vi "acquistion Real and Imaginary spectrum.vi"(4 "slope":i32(ring)=10280 items=["Rising"=10280, "Falling"=10171], 5 "maximum value":dbl=5.0, 6 "Triggering level":dbl format="%0.2f", 7 "minimum value":dbl=-5.0, 8 "error in":errorcluster, 9 "Sampling Frecuency (Hz)":dbl, 10 "Number of Samples":i32=-1, 11 "Analog In Channels":T4) -> (0 "error out":errorcluster, 3 "Data Read":waveform(dbl)[](graph))   [LabVIEW 2017]
uses:
  <vilib>/Analysis/4window.llb/windowTd.ctl
  <vilib>/DAQmx/read.llb/DAQmx Read (Analog 1D Wfm NChan NSamp).vi
  <vilib>/DAQmx/create/channels.llb/DAQmx Create Channel (AI-Voltage-Basic).vi
  <vilib>/DAQmx/configure/timing.llb/DAQmx Timing (Use Waveform).vi
  <vilib>/DAQmx/configure/trigger.llb/DAQmx Start Trigger (Analog Edge).vi
  <vilib>/DAQmx/miscellaneous.llb/DAQmx Fill In Error Info.vi
  <vilib>/measure/maspectr.llb/FFT Spectrum (Real-Im) for N Chan.vi
  <instrlib>/NI USB-6356/NI USB-6356.lvlib
  <vilib>/Analysis/NI_AALPro.lvlib
  <vilib>/measure/NI_MAPro.lvlib
panel:
  in  "window parameter":dbl=nan
  out "Real Part 2":T1(graph)
  out "Imaginary Part":T2(graph)
  in  "gain":dbl=1.0 min=1.0
  in  "Use Trigger?":bool
  out "Real Part":cluster{"f0":dbl, "df":dbl, "magnitude":dbl[]}(graph)
  out "averages completed":dbl
  out "averaging done":bool
  in  "averaging parameters":T3={"averaging mode"=enum."Vector averaging", "weighting mode"=enum."Exponential", "number of averages"=10} {"number of averages" min=1}
  in  "restart averaging (F)":bool
  in  "Channel Trigger":u16(ring) items=["ai0", "ai1", "ai2", "ai3", "ai4", "ai5", "ai6", "ai7"]
  in  "Stop Process":bool
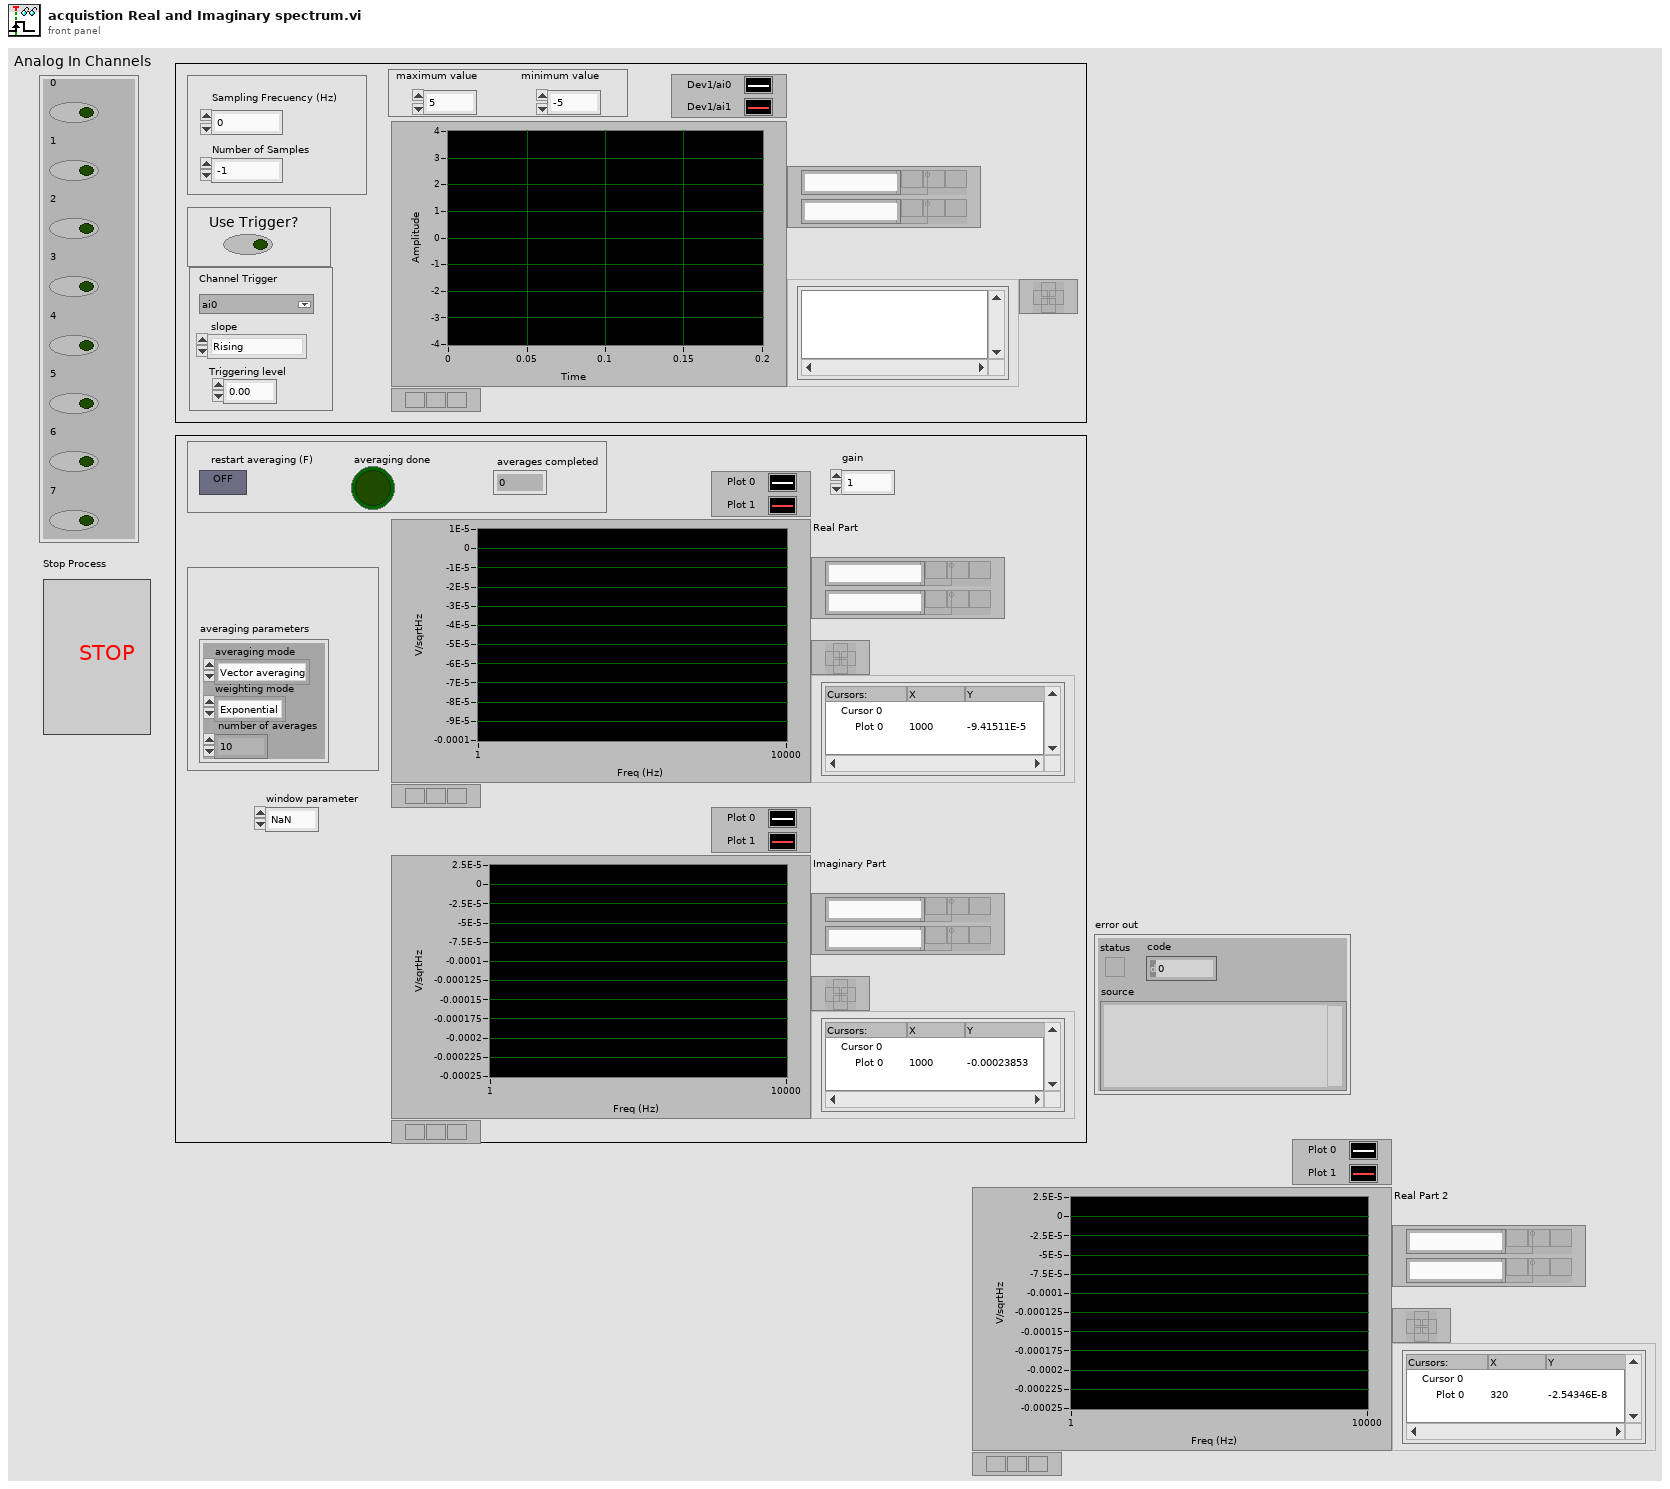
[diagram p1: front panel]
types:
  T1 = cluster{"f0":dbl, "df":dbl, "imaginary part":dbl[]}[]
  T2 = cluster{"f0":dbl, "df":dbl, "imaginary part":dbl[]}
  T3 = cluster{"averaging mode":enum16{"No averaging", "Vector averaging", "RMS averaging", "Peak hold"}, "weighting mode":enum16{"Linear", "Exponential"}, "number of averages":u32}
  T4 = cluster{"0":bool, "1":bool, "2":bool, "3":bool, "4":bool, "5":bool, "6":bool, "7":bool}
  T5 = typedef "NI_AALPro.lvlib/windowTd.ctl" = u32
  T6 = enum8{"Enabled", "Disabled", "Disabled and Grayed Out"}
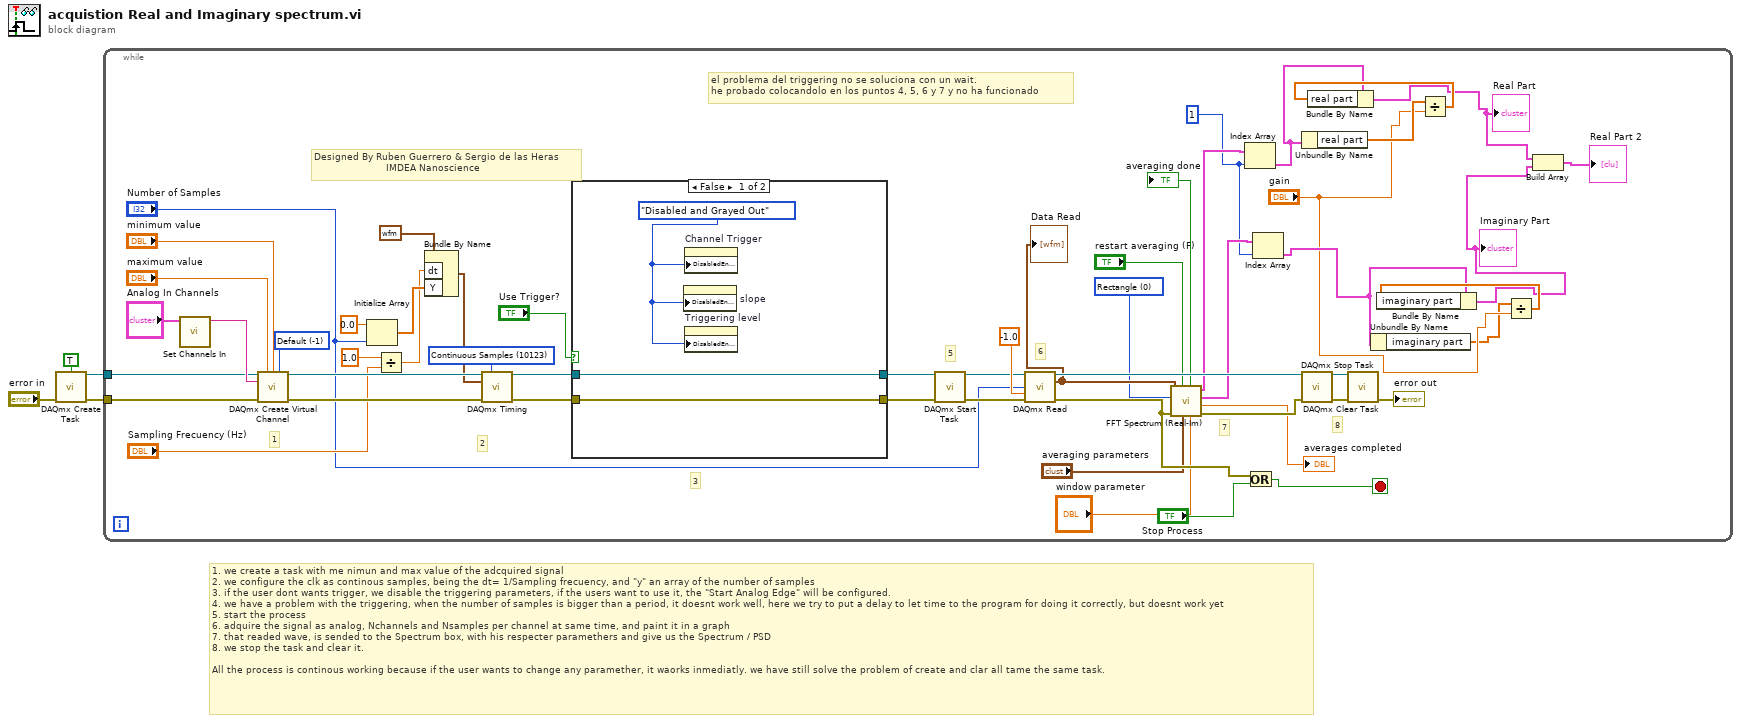
[diagram p0: block diagram]
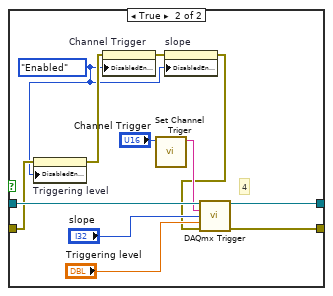
[diagram p2: hidden frame]
diagram:
  # "1. we create a task with me nimun and max value of the adcquired signal\n2. we configure the clk as continous samples, being the dt= 1/Sampling frecuency, and \"y\" an array of the number of samples\n3. if the user dont wants trigger, we disable the triggering parameters, if the users want to use it, the \"Start Analog Edge\" will be configured.\n4. we have a problem with the triggering, when the number of samples is bigger than a period, it doesnt work well, here we try to put a delay to let time to the program for doing it correctly, but doesnt work yet\n5. start the process\n6. adquire the signal as analog, Nchannels and Nsamples per channel at same time, and paint it in a graph\n7. that readed wave, is sended to the Spectrum box, with his respecter paramethers and give us the Spectrum / PSD\n8. we stop the task and clear it.\n\nAll the process is continous working because if the user wants to change any paramether, it waorks inmediatly. we have still solve the problem of create and clar all tame the same task."
  n1 = call <vilib>:"DAQmx Create Task.vi"("auto cleanup"=TRUE, "error in"="error in") -> ("task out"=w2:refnum<k21>, "error out"=w1:errorcluster)  [unwired: 12 in]
  n2 = while {
    tunnel: w2 -> [w33]
    tunnel: w1 -> [w32]
    stop <- w35 stop-if-true
    w5 = 1 ("index")
    w25 = T5 0 items=["Rectangle"=0, "Hanning"=1, "Hamming"=2, "Blackman-Harris"=3, "Exact Blackman"=4, "Blackman"=5, "Flat Top"=6, "4 Term B-Harris "=7, "7 Term B-Harris"=8, "Low Sidelobe"=9, "Blackman Nuttall"=11, "Triangle"=30, "Bartlett-Hanning"=31, "Bohman"=32, "Parzen"=33, "Welch"=34, "Kaiser"=60, "Dolph-Chebyshev"=61, "Gaussian"=62] ("window")
    w54 = 10123 items=["Finite Samples"=10178, "Continuous Samples"=10123, "Hardware Timed Single Point"=12522] ("sample mode")
    w55 = -1 items=["Default"=-1, "RSE"=10083, "Differential"=10106, "Pseudodifferential"=12529] ("output terminal configuration")
    # "el problema del triggering no se soluciona con un wait.\nhe probado colocandolo en los puntos 4, 5, 6 y 7 y no ha funcionado"
    # "8"
    # "7"
    # "6"
    # "5"
    # "3"
    # "2"
    # "1"
    # "Designed By Ruben Guerrero & Sergio de las Heras\n                        IMDEA Nanoscience"
    n3 = call <instrlib>:"Set Channels In.vi"("Analog In Channels"="Analog In Channels") -> ("String"=w47:string)  [unwired: 10 in]
    n4 = call-poly <vilib>:"DAQmx Create Virtual Channel.vi"("task in"=w33, "maximum value"="maximum value", "minimum value"="minimum value", "input terminal configuration"=w55, "physical channels"=w47, "error in"=w32) -> ("task out"=w53:refnum<k21>, "error out"=w45:errorcluster)  [unwired: 8 in]
    n5 = Initialize Array(0.0 ("element"), "Number of Samples") -> (w48:dbl[])
    n6 = Divide(x=1.0, y="Sampling Frecuency (Hz)") -> (x/y=w43:dbl)
    n7 = Bundle By Name(cluster=waveform(dbl) {"t0"=timestamp(0 s since 1904-01-01), "dt"=0.001, "Y"=array[1000 elements]} ("signal out"), "dt"=w43, "Y"=w48) -> (w41:waveform(dbl))
    n8 = call-poly <vilib>:"DAQmx Timing.vi"("task/channels in"=w53, "sample mode"=w54, "waveform"=w41, "error in"=w45) -> ("task out"=w40:refnum<k21>, "error out"=w39:errorcluster)  [unwired: 10 in]
    n9 = case shown="False" "Use Trigger?" {
      tunnel: w40 -> [w61 w73]
      tunnel: w39 -> [w60 w66]
      tunnel: [w61 w72] -> w28
      tunnel: [w60 w71] -> w27
      frame False {
        w59 = T6."Disabled and Grayed Out" ("Disabled")
        n10 = property on="slope" class="Ring (strict)"("DisabledEnum"=w59) -> ()  [unwired: 2 in, 2 out]
        n11 = property on="Channel Trigger" class="Ring (strict)"("DisabledEnum"=w59) -> ()  [unwired: 2 in, 2 out]
        n12 = property on="Triggering level" class="DigNum (strict)"("DisabledEnum"=w59) -> ()  [unwired: 2 in, 2 out]
      }
      frame True {
        w62 = T6."Enabled" ("Disabled")
        # "4"
        n13 = property on="Triggering level" class="DigNum (strict)"(error in=w66, "DisabledEnum"=w62) -> (error out=w65:errorcluster)  [unwired: 1 in, 1 out]
        n14 = property on="Channel Trigger" class="Ring (strict)"(error in=w65, "DisabledEnum"=w62) -> (error out=w64:errorcluster)  [unwired: 1 in, 1 out]
        n15 = call <instrlib>:"Set Channel Triger.vi"("Channel Trigger"="Channel Trigger") -> ("String Channel"=w69:string)  [unwired: 10 in]
        n16 = property on="slope" class="Ring (strict)"(error in=w64, "DisabledEnum"=w62) -> (error out=w63:errorcluster)  [unwired: 1 in, 1 out]
        n17 = call-poly <vilib>:"DAQmx Trigger.vi"("task/channels in"=w73, "source"=w69, "slope"="slope", "level"="Triggering level", "error in"=w63) -> ("task out"=w72:refnum<k21>, "error out"=w71:errorcluster)  [unwired: 9 in]
      }
    }
    n18 = call <vilib>:"DAQmx Start Task.vi"("task/channels in"=w28, "error in"=w27) -> ("task out"=w31:refnum<k21>, "error out"=w30:errorcluster)  [unwired: 12 in]
    n19 = call-poly <vilib>:"DAQmx Read.vi"("task/channels in"=w31, "number of samples per channel"="Number of Samples", "timeout"=-1.0, "error in"=w30) -> ("task out"=w38:refnum<k21>, "data"=w26:waveform(dbl)[], "error out"=w24:errorcluster)  [unwired: 9 in]
    "Data Read" <- w26
    n20 = call-poly <vilib>:"FFT Spectrum (Real-Im).vi"("window parameter"="window parameter", "averaging parameters"="averaging parameters", "restart averaging (F)"="restart averaging (F)", "error in (no error)"=w24, "window"=w25, "time signals"=w26) -> ("error out"=w23:errorcluster, "averages completed"=→"averages completed":dbl, "imaginary parts"=w17:T1, "real parts"=w19:cluster{"f0":dbl, "df":dbl, "real part":dbl[]}[], "averaging done"=→"averaging done":bool)  [unwired: 1 in]
    n21 = Index Array(array=w19, index=w5) -> (element=w13:cluster{"f0":dbl, "df":dbl, "real part":dbl[]})
    n22 = Or(x=w24, y="Stop Process") -> (x .or. y?=w35:bool)
    n23 = Index Array(array=w17, index=w5) -> (element=w9:T2)
    n24 = Unbundle By Name(w13) -> ("real part"=w10:dbl[])
    n25 = call <vilib>:"DAQmx Stop Task.vi"("task/channels in"=w38, "error in"=w23) -> ("task out"=w51:refnum<k21>, "error out"=w52:errorcluster)  [unwired: 12 in]
    n26 = call <vilib>:"DAQmx Clear Task.vi"("task in"=w51, "error in"=w52) -> ("error out"=→"error out":errorcluster)  [unwired: 13 in]
    n27 = Unbundle By Name(w9) -> ("imaginary part"=w6:dbl[])
    n28 = Divide(x=w10, y="gain") -> (x/y=w14:dbl[])
    n29 = Bundle By Name(cluster=w13, "real part"=w14) -> (w12:cluster{"f0":dbl, "df":dbl, "real part":dbl[]})
    "Real Part" <- w12
    n30 = Divide(x=w6, y="gain") -> (x/y=w11:dbl[])
    n31 = Bundle By Name(cluster=w9, "imaginary part"=w11) -> (w7:T2)
    "Imaginary Part" <- w7
    n32 = Build Array(w12, w7) -> (→"Real Part 2":T1)
  }
